vi "PH_Strings.Remove trailing Zeros.vi"(1 "Input String":string) -> (0 "Output String":string)   [LabVIEW 2014, in "PH_Common.lvlib"]
doc: "If the input string contains \"\\OO\", the text BEFORE is the output string; else: the output equals the input."
uses:
  PH_Common.lvlib
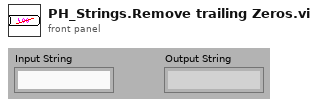
[diagram p1: front panel]
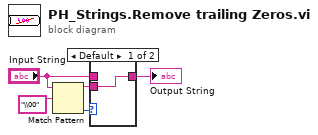
[diagram p0: block diagram]
diagram:
  n1 = Match Pattern(string="Input String", regular expression="\\00" ("search string")) -> (before substring=w2:string, offset past match=w1:i32)  [unwired: 1 in, 2 out]
  n2 = case shown="Default" w1 {
    tunnel: [w6 w7] -> w5
    tunnel: "Input String" -> [_ w7]
    tunnel: w2 -> [w6 _]
    frame Default {
    }
    frame -1 {
    }
  }
  "Output String" <- w5
